vi "FY6900_Load.vi"() -> ()   [LabVIEW 2020]
panel:
  in  "Port3":string(combo)
  in  "Port2":string(combo)
  in  "Port1":string(combo)
  in  "Wave":string(combo)
  in  "stop":bool
  in  "Load to AWGs":bool
  in  "ÀFrequency":dbl
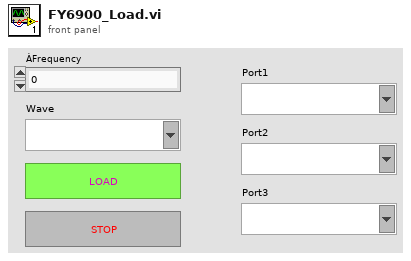
[diagram p1: front panel]
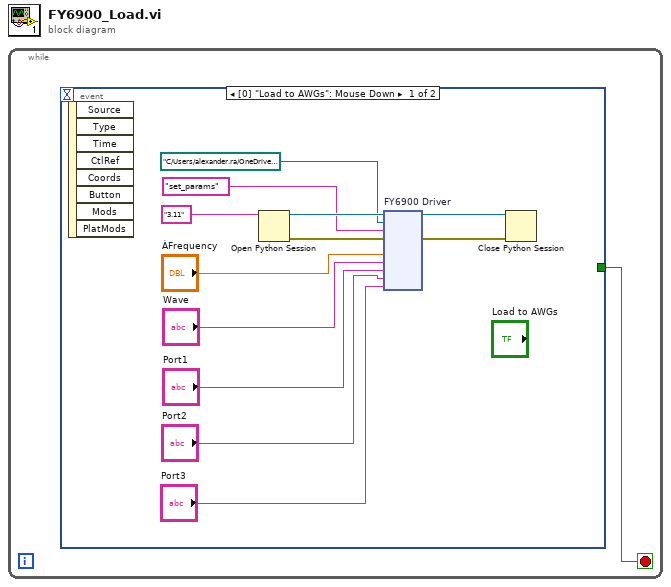
[diagram p0: block diagram]
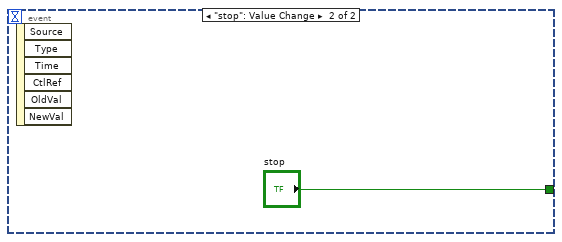
[diagram p2: hidden frame]
diagram:
  n1 = while {
    stop <- w1 stop-if-true
    n2 = event shown="[0] \"Load to AWGs\": Mouse Down" {
      selector: _ -> [_ _]
      dyn-events: _ -> [_ _]
      timeout: _ -> [_ _]
      tunnel: [_ "stop"] -> w1
      event "Load to AWGs": Mouse Down {
        n3 = event-data() -> ()  [unwired: 1 in, 8 out]
        n4 = Open Python Session(python version="3.11" ("Python version")) -> (session out=w13:refnum<k35>, error out=w11:errorcluster)  [unwired: 2 in]
        n5 = node "FY6900 Driver"(w13, path "C:/Users/alexander.ra/OneDrive - Technion/Documents/fy6900/fygenmidware.py" ("module path"), "set_params" ("function name"), w11, "ÀFrequency", "Wave", "Port1", "Port2", "Port3") -> (w12:refnum<k35>, w10:errorcluster)  [unwired: 7 in, 2 out]
        n6 = Close Python Session(session in=w12, error in=w10) -> ()  [unwired: 1 out]
      }
      event "stop": Value Change {
        n7 = event-data() -> ()  [unwired: 1 in, 6 out]
      }
    }
  }
